vi "Init.vi"(8 "Error In":errorcluster) -> (0 "Error Out":errorcluster, 3 "Message Queues":T1)   [LabVIEW 2017, in "Client.lvlib" / "CommsFrameWork.lvlib"]
uses:
  CommsFrameWork.lvlib
  TypeDefs/CommReferences.ctl
  ServerLib/SubLibs/Message Queue/MessageCluster.ctl
  EnqueueMessage(Single).vi
  ClientErrorHandler/ClientErrorHandler.lvlib
  ServerLib/SubLibs/Message Queue/Message Queue.lvlib
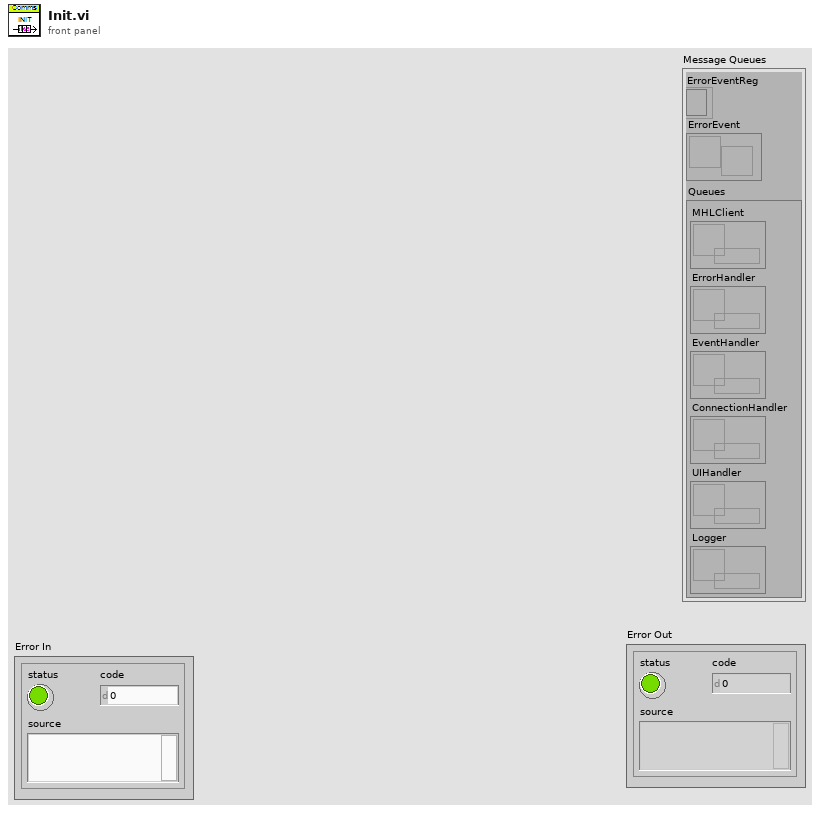
[diagram p1: front panel]
types:
  T1 = typedef "Client.lvlib/CommsFrameWork.lvlib/CommReferences.ctl" = cluster{"ErrorEventReg":refnum<event-registration>, "ErrorEvent":refnum<user-event>, "Queues":cluster{"MHLClient":refnum<queue>, "ErrorHandler":refnum<queue>, "EventHandler":refnum<queue>, "ConnectionHandler":refnum<queue>, "UIHandler":refnum<queue>, "Logger":refnum<queue>}}
  T2 = typedef "Client.lvlib/CommsFrameWork.lvlib/InternalData.ctl" = cluster{"Connection Data":cluster{"IP":string, "Port":string, "ClientName":string}}
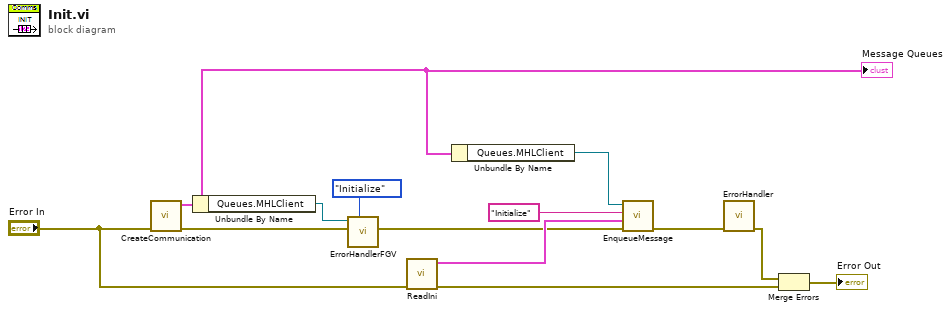
[diagram p0: block diagram]
diagram:
  n1 = call "CreateCommunication.vi"("error in (no error)"="Error In") -> ("error out"=w2:errorcluster, "Message Queues"=w12:T1)  [unwired: 9 in]
  "Message Queues" <- w12
  n2 = Unbundle By Name(w12) -> ("Queues.MHLClient"=w3:refnum<queue>)
  n3 = call "ErrorHandlerFGV.vi"("Command(CheckErrors)"=enum16{"Initialize", "CheckErrors"}."Initialize", "Error In"=w2, "MHL"=w3) -> ("Error Out"=w1:errorcluster)  [unwired: 8 in]
  n4 = call "ReadIni.vi"("Error In"="Error In") -> ("Error Out"=w8:errorcluster, "InternalData"=w9:T2)  [unwired: 9 in]
  n5 = Unbundle By Name(w12) -> ("Queues.MHLClient"=w13:refnum<queue>)
  n6 = call-poly "EnqueueMessage.vi"("error in (no error)"=w1, "Message Data"=w9, "Message"="Initialize", "Message Queue"=w13) -> ("error out"=w6:errorcluster)  [unwired: 6 in, 1 out]
  n7 = call "ErrorHandler.vi"("error in (no error)"=w6) -> ("error out"=w5:errorcluster)  [unwired: 10 in]
  n8 = Merge Errors(w5, w8) -> (→"Error Out":errorcluster)
